vi "PI Controller.vi"(6 "Ti":dbl, 7 "Ts":dbl, 9 "Kp":dbl, 10 "yk":dbl, 11 "rk":dbl) -> (3 "Control signal":dbl)   [LabVIEW 2025]
panel:
  out "ek1":dbl
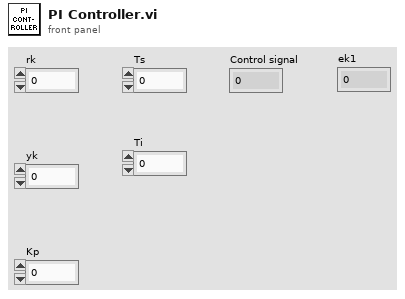
[diagram p1: front panel]
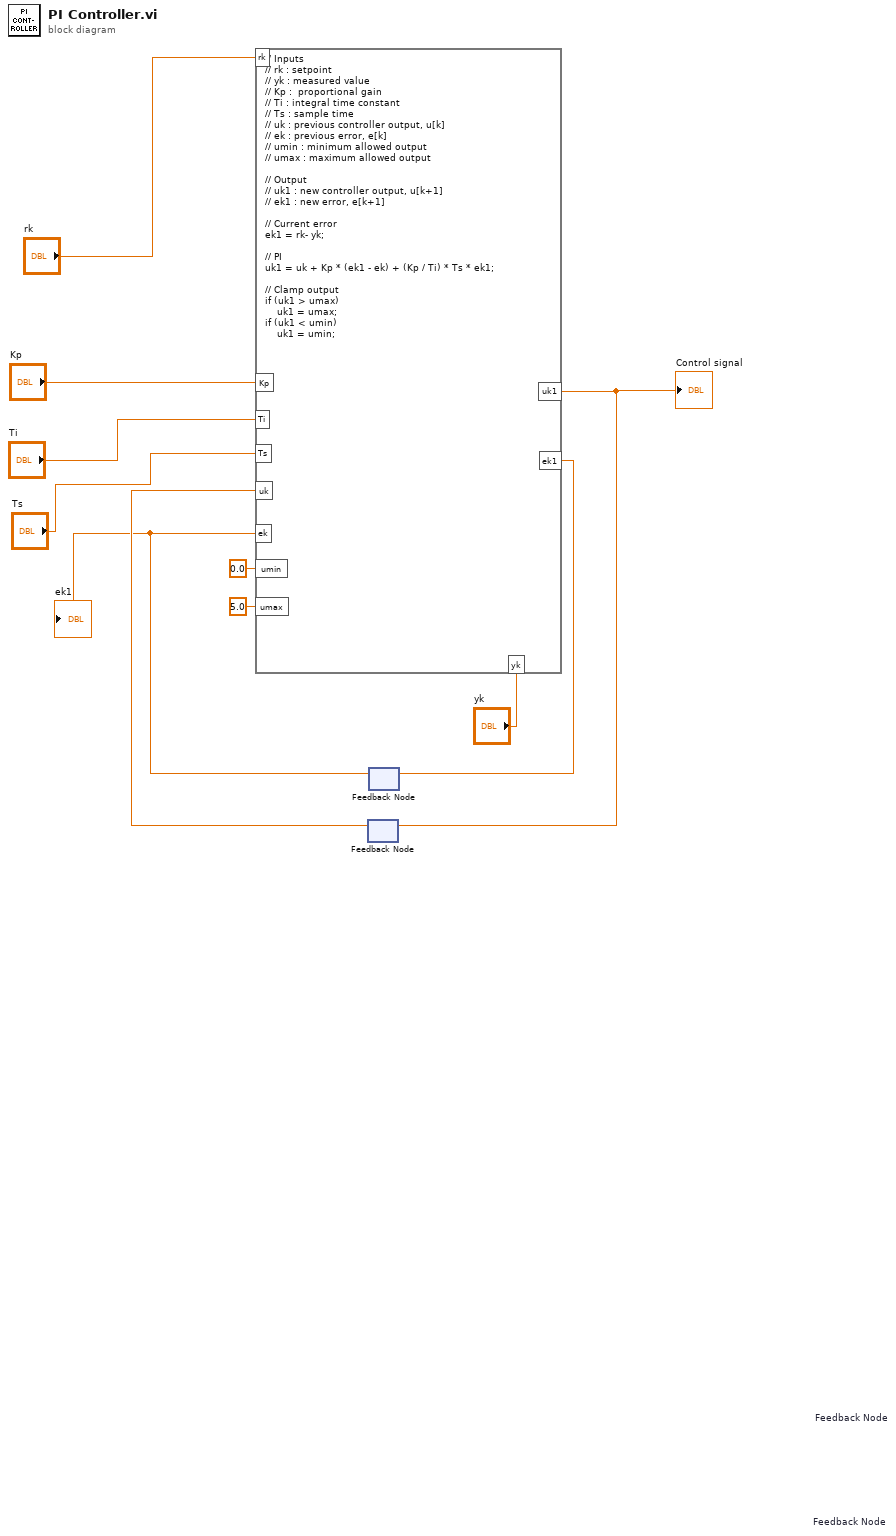
[diagram p0: block diagram]
diagram:
  n1 = feedback #1 "Feedback Node"() -> (w7:dbl)  [unwired: 1 in]
  n2 = feedback #2 "Feedback Node"() -> (w5:dbl)  [unwired: 1 in]
  "ek1" <- w5
  n3 = formula code="// Inputs\n// rk : setpoint\n// yk : measured value\n// Kp :  proportional gain\n// Ti : integral time constant\n// Ts : sample time\n// uk : previous controller output, u[k]\n// ek : previous error, e[k]\n// umin : minimum allowed output\n// umax : maximum allowed output\n\n// Output\n// uk1 : new controller output, u[k+1]\n// ek1 : new error, e[k+1]\n\n// Current error\nek1 = rk- yk;\n\n// PI \nuk1 = uk + Kp * (ek1 - ek) + (Kp / Ti) * Ts * ek1;\n\n// Clamp output\nif (uk1 > umax)\n    uk1 = umax;\nif (uk1 < umin)\n    uk1 = umin;"("rk"="rk", "yk"="yk", "Kp"="Kp", "Ti"="Ti", "Ts"="Ts", "uk"=w7, "ek"=w5, "umin"=0.0 ("input variable"), "umax"=5.0 ("input variable")) -> ("uk1"=w6:dbl, "ek1"=w4:dbl)
  "Control signal" <- w6
  n4 = feedback-in #1(w6) -> ()
  n5 = feedback-in #2(w4) -> ()
